vi "simulate regional.vi"(2 "liability?  (benefit)":bool, 3 "estimated team value data":path, 4 "source data":path) -> (0 "Array":i16[][](array[numeric]), 1 "correct # of elements in source data file?":bool)   [LabVIEW 2009]
uses:
  <vilib>/Utility/file.llb/Read From Spreadsheet File (I64).vi
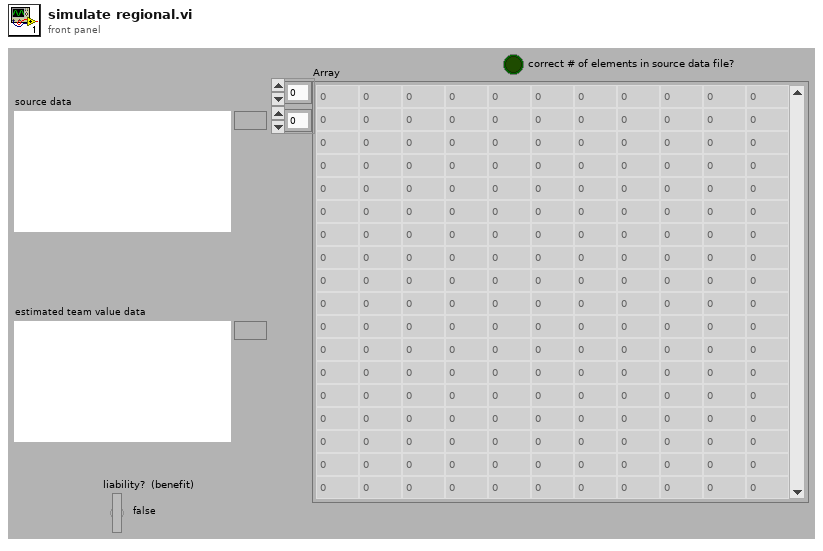
[diagram p1: front panel]
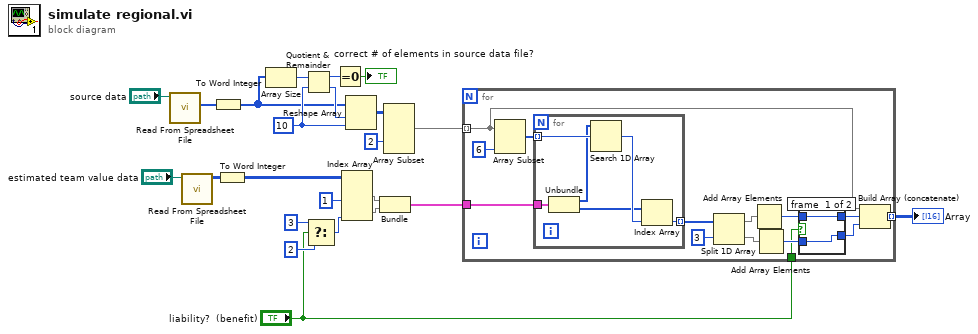
[diagram p0: block diagram]
diagram:
  w19 = 10 ("dimension size")
  n1 = call-poly <vilib>:"Read From Spreadsheet File.vi"("file path (dialog if empty)"="source data") -> ("first row"=w10:i64[])  [unwired: 6 in, 4 out]
  n2 = call-poly <vilib>:"Read From Spreadsheet File.vi"("file path (dialog if empty)"="estimated team value data") -> ("all rows"=w6:i64[][])  [unwired: 6 in, 4 out]
  n3 = To Word Integer(number=w10) -> (16bit integer=w9:i16[])
  n4 = To Word Integer(number=w6) -> (16bit integer=w5:i16[][])
  n5 = Array Size(array=w9) -> (size(s)=w20:i32)
  n6 = Quotient & Remainder(x=w20, y=w19) -> (x-y*floor(x/y)=w17:i32, floor(x/y)=w18:i32)
  n7 = Select(t=3 ("index (col)"), s="liability?  (benefit)", f=2 ("index (col)")) -> (s? t:f=w2:i32)
  n8 = Equal To 0?(x=w17) -> (x = 0?=→"correct # of elements in source data file?":bool)
  n9 = Index Array(array=w5, index (col) #1=1 ("disabled index (col)"), index (col) #2=w2) -> (element #1=w22:i16[], element #2=w21:i16[])  [unwired: 2 in]
  n10 = Reshape Array(w9, w18, w19) -> (w15:i16[][])
  n11 = Bundle(w22, w21) -> (w12:cluster{i16[], i16[]})  [unwired: 1 in]
  n12 = Array Subset(array=w15, index (col)=2 ("index")) -> (w13:i16[][])  [unwired: 3 in]
  n13 = for {
    tunnel: w13 -> [w30] mode=indexing
    tunnel: w12 -> [w36]
    tunnel: [w29] -> w11 mode=indexing
    tunnel: "liability?  (benefit)" -> [w24]
    n14 = Array Subset(array=w30, length=6) -> (w35:i16[])  [unwired: 1 in]
    n15 = for {
      tunnel: w36 -> [w46]
      tunnel: w35 -> [w47] mode=indexing
      tunnel: [w42] -> w34 mode=indexing
      n16 = Unbundle(w46) -> (w45:i16[], w43:i16[])
      n17 = Search 1D Array(1D array=w45, element=w47) -> (index of element=w44:i32)  [unwired: 1 in]
      n18 = Index Array(array=w43, index=w44) -> (element=w42:i16)
    }
    n19 = Split 1D Array(array=w34, index=3) -> (first subarray=w32:i16[], second subarray=w31:i16[])
    n20 = Add Array Elements(numeric array=w32) -> (sum=w27:i16)
    n21 = Add Array Elements(numeric array=w31) -> (sum=w25:i16)
    n22 = case shown="True" w24 {
      tunnel: [w39 w40] -> w28
      tunnel: w27 -> [w39 w41]
      tunnel: [w38 w41] -> w26
      tunnel: w25 -> [w38 w40]
      frame #0 {
      }
      frame #1 {
      }
    }
    n23 = Build Array (concatenate)(w30, w28, w26) -> (w29:i16[])
  }
  "Array" <- w11
